vi "XLP80_Globals_Status.vi"() -> ()   [LabVIEW 2021]
uses:
  XLP80_Action/XLP80_Action_TDefEnumControl.ctl
panel:
  in  "AlarmsTab":T1(tab)
  in  "Read DI":bool
  in  "ChartData":sgl[][](array[numeric])
  in  "Control":T2
  in  "H31_OTV_Logic":bool
  out "Mode GUI":refnum<vi>
  out "SYS_Error_Code":u32 format="%.0x"
  out "LogIndex":i32[](array[numeric])
  in  "PW":string="Augsburg123"
  out "CVM":sgl[](array[numeric])
  out "DeviceServer":bool
  out "ErrorMessage":string[](array[string])=["No Error", "C01_RF Diagnosis Pin", "A03_ETC Degraded pr Blocked", "A03_ETC <0rpm or >280.000rpm", "A03 ETC Warning Code", "A03 ETC Error Code", "A03 ETC Power > 3500W", "A03 ETC ConverterTemp > 100°C", "A03_ETC PT100Temp >100°C", "A03_ETC THCTemp >100°C", "A03_ETC GasBearing <50", "C04_DI Temp >80°C", "C06_ET Full", "C07_B Error", "C07_B BoardTemp <0°C or >45°C", "C07_B Current>3200A", "C07_B Voltage <70V or", "C07_B MaxCellTemp <0°C or >45°C", "C07_B MinCellTemp <0°C or >45°C", "C07_B SOC <10%", "C07_B SOH <90%", "C07_B PreWarn SOC", "C07_B PreWarn Curr High", "C07_B PreWarn Volt High/Low", "C07 PreWarn Temp", "C07_B BatError Intern", "C07_B BatError DataValid", "C07_B BatError Volt", "C07_B BatError Temp", "C07_B CECUError Intern", "C07_B CECUError Current", "C07_B CECUError Volt", "C07_B CECUError Temp", "C07_B CECUError Comm", "C07_B CECUError Supply", "C07_B CECUError Reserved", "C07_B CECUError Service", "C08_AMB Temp <0°C or > 45°C", "C08_AMB Press <90kPa or >110kPa", "A11_HBV Position", "A12_SIV Position", "A13_SOV Position", "A14_HFM Temp >50°C", "H31_OTV Press <20bar or >350bar", "H31_OTV Temp >100°C", "H36_GHU StartupPress1 Timeout", "H36_GHU StartupPress2 Timeout", "H42_HRB SysState Error", "H42_HRB MtrNTCFlr_DrCnd", "H42_HRB MTtr_Temp_Err", "H42_HRB Mtr_Temp_DrCnd", "H42_HRB BrdgDrv_VCC_UV_Err", "H42_HRB ShortToGround_Err", "H42_HRB ShortToBat_Err", "H42_HRB E2E_Err", "H42_HRB SpdLimitRq_Err", "H42_HRB Blocked_Err", "H42_HRBBatt_Vltg_Err", "H42_HRB ECU_Temp_Err", "H42_HRB ECU_Temp_DrCnd", "H42_HRB KNF Error", "H42_WT Tank Full", "H51_STK LowCellVolt <200mV", "H51_STK TotalVolt <31V or >75V", "H51_STK Startup CellVolt Timeout", "H51_STK Shutdown CellVolt Timeout", "H53_PV Startup Timeout", "C54_SI Temp >80°C", "H55_SI Press >2,5bar", "H62_HLD ErrorCode = 3", "H62_HLD Concentration >122.500ppm", "H63_HLD ErrorCode = 3", "H63_HLD Concentration >122.500ppm", "E71_DCDC Precharge", "E71_DCDC Operational", "E74_ISO R <0kOhm", "E74_ISO IsoError", "E74_ISO Err Chassis", "E74_ISO Sysstoer", "E74_ISO IsoWarn"]
  out "S91_SYS_Error_Code":u32[](array[numeric])=[0, 1, 2, 3, 4, 5, 6, 7, 8, 9, 10, 11, 12, 13, 14, 15, 16, 17, 18, 19, 20, 21, 22, 23, 24, 25, 26, 27, 28, 29, 30, 31, 32, 33, 34, 35, 36, 37, 38, 39, 40, 41, 42, 43, 44, 45, 46, 47, 48, 49, 50, 51, 52, 53, 54, 55, 56, 57, 58, 59, 60, 61, 62, 63, 64, 65, 66, 67, 68, 69, 70, 71, 72, 73, 74, 75, 76, 77, 78, 79] format="%.0x"
  out "data":path
  out "DynamicVIs":path
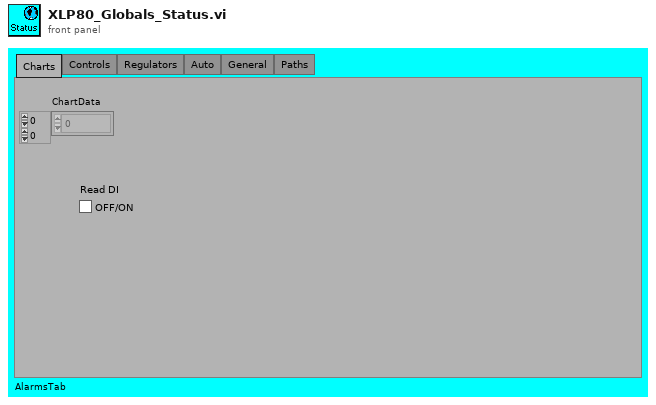
[diagram p1: front panel]
types:
  T1 = enum32{"Charts", "Controls", "Regulators", "Auto", "General", "Paths"}
  T2 = typedef "XLP80_Action_TDefEnumControl.ctl" = enum16{"Testmode_A", "Testmode_B"}
diagram:
